vi "Soft_Robot_Model2.vi"() -> ()   [LabVIEW 2015]
uses:
  <vilib>/addons/Control Design/_Model Construction/Model Typedefs.llb/CD State Space Model (MIMO).ctl
  <vilib>/addons/Control Design/_Model Construction/Model Typedefs.llb/CD General Elements.ctl
  <vilib>/Platform/TimedLoop/XDataNode/timing_clust.ctl
  <vilib>/Platform/TimedLoop/XDataNode/nitl_modes.ctl
  <vilib>/Platform/TimedLoop/XDataNode/wakeup.ctl
  <vilib>/addons/Control Design/_Stochastic Systems/Stochastic Systems.llb/Stochastic Systems SubVIs/cd_Stochastic State-Space Model.ctl
  <vilib>/addons/Control Design/_Stochastic Systems/Stochastic Systems.llb/Stochastic Systems SubVIs/cd_Second-Order Statistics Noise Model.ctl
  <vilib>/addons/Control Design/_Model Construction/Model Creation.llb/Model Creation SubVI/cd_Create State Space Model.vi
  <vilib>/Simulation/Estimation/Implementation/NILVSim Discrete Kalman Filter.llb/SIM Disc KF Pred and Corr with Pred Gain with Checking Direct LV.vi
  <vilib>/addons/Control Design/_Implementation/CD State Feedback Controller (Multiple Outputs).vi
  <vilib>/FPGAPlugInAG/myRIO-1900/niLvFpga_Open_myRIO-1900.vi
  <vilib>/rvi/interface/common/dynamic/niFpgaDynamicAddResources.vi
  <vilib>/Utility/error.llb/Error Cluster From Error Code.vi
  <vilib>/rvi/errors/niLvFpgaAdjustHostInterfaceError.vi
  <vilib>/FPGAPlugInAG/Dynamic/niLvFpga_Close_Dynamic.vi
  <vilib>/Simulation/Implementation/XNodeFramework/SimXNode/SimX.xnode
  <vilib>/rvi/interface/nirviOpenFPGA/nirviOpenFPGA.xnode
  FPGA Bitfiles/ACC20115_FPGATarget_CurrentControlle_Dt5vFgOzYtY.lvbitx
  Current Controller.vi
  <vilib>/Platform/TimedLoop/XDataNode/XDataNode.xnode
  <vilib>/rvi/interface/nirviReadWriteControl/nirviReadWriteControl.xnode
  <vilib>/rvi/interface/nirviCloseFPGA/nirviCloseFPGA.xnode
  <vilib>/addons/Control Design/_Model Construction/NI_LinSys_Model Creation.lvlib
  <vilib>/Platform/TimedLoop/XDataNode/XDNodeRunTimeDep.lvlib
  NiFpgaLv.dll
  <vilib>/rvi/interface/Simulation/niFpgaSimulationCallBeginRW.vi
  <vilib>/addons/Control Design/_Implementation/NI_CD_Implementation.lvlib
  <vilib>/addons/Control Design/_Stochastic Systems/NI_CD_Stochastic Systems.lvlib
  <vilib>/addons/Control Design/_Model Construction/NI_LinSys_Model Typedefs.lvlib
panel:
  in  "SP":dbl(slide) scale=0.0..100.0
  in  "Tab Control":enum32{"Outputs", "Inputs"}(tab)
  out "Fusion Data":dbl(graph)
  out "KF Post":dbl[](graph)
  in  "Stop":bool
  out "DAC Inlet Valve 2":i32(graph)
  in  "Current (mA)":i32
  out "Status?":bool
  out "State-Space Model":T1={"properties"={"Model name"="", "Input names"=[], "Output names"=[], "Input Delays"=[], "Output Delays"=[], "Sampling Time"=0.0, "Notes"=""}, "A"=[], "B"=[[3.03e-07], [4.04e-07]], "C"=[], "D"=[], "StateNames"=[], "Transport Delay"=[]} {"Transport Delay" format="%.2f"; "D" format="%#.2g"; "C" format="%#.2g"; "B" format="%#.2g"; "A" format="%#.2g"; "properties"."Sampling Time" format="%#.6p"; "properties"."Output Delays" format="%.4f"; "properties"."Input Delays" format="%.4f"}
  out "KF Gain M(k)":dbl[][](array[numeric])
  in  "A":dbl[][](array[numeric])=[[1.01, -0.1716], [0.001556, 0.9782]] format="%#.5g"
  in  "B":dbl[][](array[numeric]) format="%#.5g"
  in  "C":dbl[][](array[numeric])=[[1.089, -0.03769]] format="%#.5g"
  out "error out":errorcluster
  out "KF Error":errorcluster
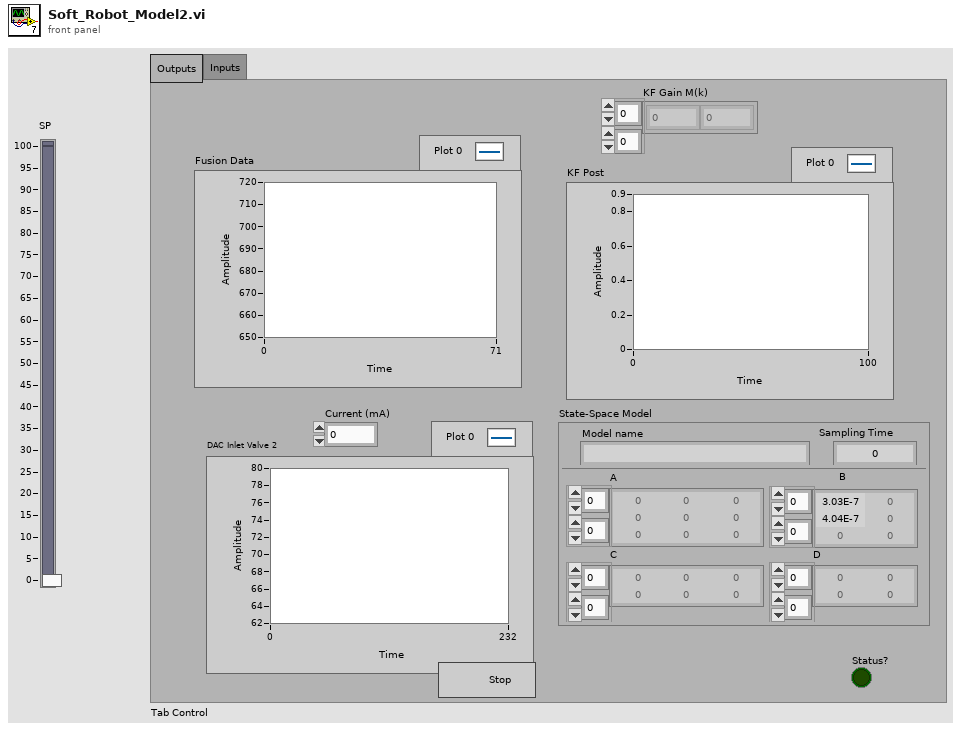
[diagram p1: front panel]
types:
  T1 = typedef "NI_LinSys_Model Typedefs.lvlib/CD State Space Model (MIMO).ctl" = cluster{"properties":T2, "A":dbl[][], "B":dbl[][], "C":dbl[][], "D":dbl[][], "StateNames":string[], "Transport Delay":dbl[][]}
  T2 = typedef "NI_LinSys_Model Typedefs.lvlib/CD General Elements.ctl" = cluster{"Model name":string, "Input names":string[], "Output names":string[], "Input Delays":dbl[], "Output Delays":dbl[], "Sampling Time":dbl, "Notes":string}
  T3 = typedef "NI_CD_Stochastic Systems.lvlib/cd_Second-Order Statistics Noise Model.ctl" = cluster{"Q":dbl[][], "E{w}":dbl[], "E{v}":dbl[], "R":dbl[][], "N":dbl[][]}
  T4 = typedef "NI_CD_Stochastic Systems.lvlib/cd_Stochastic State-Space Model.ctl" = cluster{"Sampling Time (s)":dbl, "G":dbl[][], "B":dbl[][], "A":dbl[][], "C":dbl[][], "D":dbl[][], "H":dbl[][]}
  T5 = typedef "XDNodeRunTimeDep.lvlib/timing_clust.ctl" = cluster{"Expected End [f-1]":u64, "Actual End [f-1]":u64, "Finished Late? [f-1]":bool, "Expected End [i-1]":u64, "Actual End [i-1]":u64, "Finished Late? [i-1]":bool, "Expected Start [i]":u64, "Actual Start [i]":u64, "Expected Start [f]":u64, "Actual Start [f]":u64, "Source Name":string, "Structure Name":string, "Period":i64, "Deadline":i64, "Offset":i64, "Start":i64, "Priority":i32, "Timeout":i32, "Mode":T6, "Wakeup Reason":T7, "Error":errorcluster, "Source Type":string, "Secondary Source Type":string, "Global End Time":u64, "Global Start Time":u64, "Frame Duration":u64, "Iteration Duration":u64, "Assigned CPU":i32, "I/O Scan Engine Mode":u32}
  T6 = typedef "XDNodeRunTimeDep.lvlib/nitl_modes.ctl" = enum32{"No Change", "Process missed periods, maintain original phase", "Discard missed periods, maintain original phase", "Process missed periods, ignore original phase", "Discard missed periods, ignore original phase"}
  T7 = typedef "XDNodeRunTimeDep.lvlib/wakeup.ctl" = enum32{"Normal", "Aborted", "Asynchronous wakeup", "Timing source error", "Timed loop error", "Timeout"}
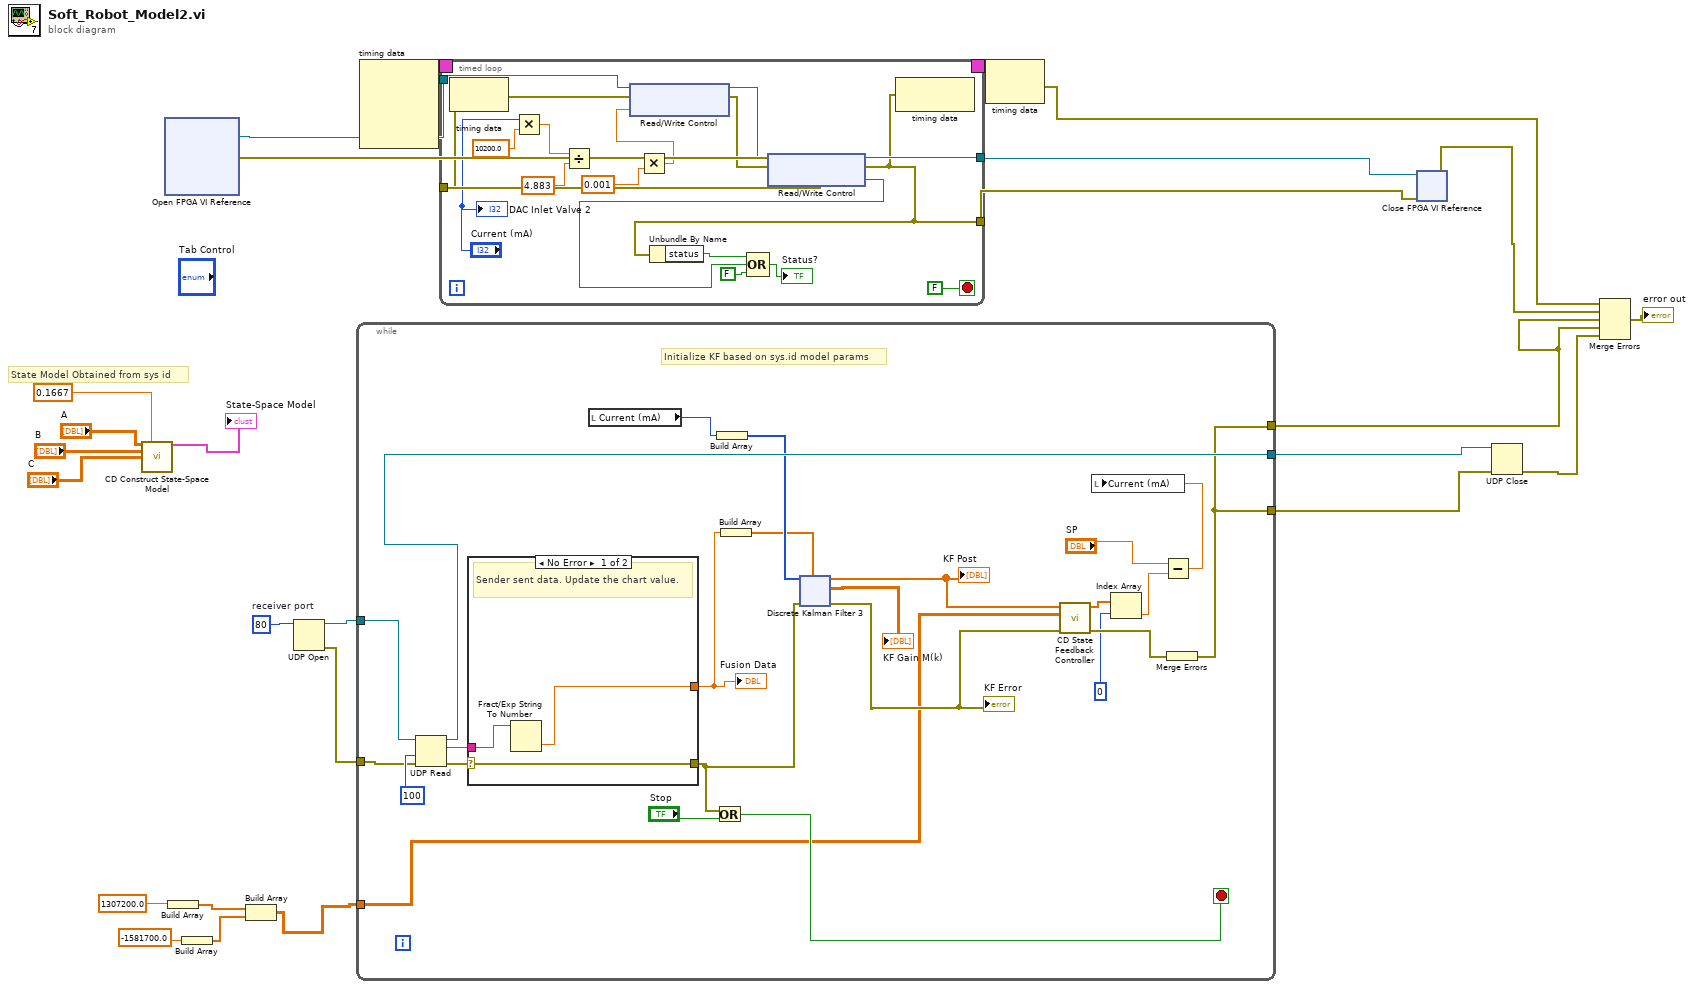
[diagram p0: block diagram]
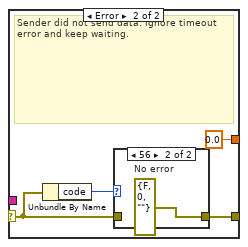
[diagram p2: hidden frame]
diagram:
  w25 = u16 80  # receiver port
  # "State Model Obtained from sys id"
  n1 = call-poly <vilib>:"CD Construct State-Space Model.vi"("A"="A", "Sampling Time (s)"=0.1667, "B"="B", "C"="C") -> ("State-Space Model"=→"State-Space Model":T1)  [unwired: 10 in, 1 out]
  n2 = xnode "Open FPGA VI Reference"() -> ("FPGA VI Reference Out"=w20:refnum<k20>, "error out"=w19:errorcluster)  [unwired: 2 in]
  n3 = Build Array(1307200.0 ("element")) -> (w4:dbl[])
  n4 = Build Array(-1581700.0 ("element")) -> (w3:dbl[])
  n5 = Build Array(w4, w3) -> (w2:dbl[][])
  n6 = UDP Open(11:w25) -> (port=w24:refnum<k16>, 0:w23:errorcluster)  [unwired: 4 in, 1 out]
  n7 = while {
    tunnel: [w33] -> w1
    tunnel: w24 -> [w45]
    tunnel: w23 -> [w44]
    tunnel: [w42] -> w22
    tunnel: [w33] -> w16
    tunnel: w2 -> [w32]
    stop <- w43 stop-if-true
    # "Initialize KF based on sys.id model params"
    n8 = UDP Read(connection ID=w45, timeout ms (25000)=100, 8:w44) -> (data out=w47:string, error out=w46:errorcluster, 3:w42:refnum<k16>)  [unwired: 3 out]
    n9 = case shown="No Error" w46 {
      selector: w46 -> [w52 w56]
      tunnel: w47 -> [w53 _]
      tunnel: [w52 w55] -> w27
      tunnel: [w51 0.0] -> w37
      frame No Error {
        # "Sender sent data. Update the chart value."
        n10 = Fract/Exp String To Number(string=w53) -> (number=w51:dbl)  [unwired: 3 in, 1 out]
      }
      frame Error {
        # "Sender did not send data. Ignore timeout error and keep waiting."
        n11 = Unbundle By Name(w56) -> ("code"=w57:i32)
        n12 = case shown="56" w57 {
          tunnel: w56 -> [w58 _]
          tunnel: [w58 w59] -> w55
          frame Default {
          }
          frame 56 {
            w59 = errorcluster {"status"=FALSE, "code"=0, "source"=""}  # No error
          }
        }
      }
    }
    "Fusion Data" <- w37
    n13 = local read "Current (mA)"() -> (w50:i32)
    n14 = Or(x=w27, y="Stop") -> (x .or. y?=w43:bool)
    n15 = Build Array ("Build Array 5")(w50) -> (w38:i32[])
    n16 = Build Array ("Build Array 6")(w37) -> (w36:dbl[])
    n17 = xnode ("Discrete Kalman Filter 3")("input u(k)"=w38, "Output y(k)"=w36, "error in (no error)"=w27) -> ("Corrected State Estimate xhat(k|k)"=w28:dbl[], "Kalman Filter Gain M(k)"=→"KF Gain M(k)":dbl[][], "error out"=w39:errorcluster)  [unwired: 5 out]
    "KF Post" <- w28
    "KF Error" <- w39
    n18 = call-poly <vilib>:"CD State Feedback Controller.vi"("error in (no error)"=w39, "Controller Gain"=w32, "States"=w28) -> ("error out"=w40:errorcluster, "Controller Action"=w35:dbl[])  [unwired: 7 in]
    n19 = Index Array(array=w35, index=0) -> (element=w31:dbl)
    n20 = Subtract(x="SP", y=w31) -> (x-y=w30:dbl)
    n21 = local write "Current (mA)"(w30) -> ()
    n22 = Merge Errors(w40) -> (w33:errorcluster)
  }
  n23 = node-c288() -> (w18:T5)  [unwired: 4 in]
  n24 = timed-loop {
    tunnel: w20 -> [w92]
    tunnel: w19 -> [w77]
    tunnel: [w76] -> w10
    tunnel: [w85] -> w26
    timing: w18 -> [_]
    timing-out: [_] -> w17
    stop <- FALSE stop-if-true
    n25 = node-c288() -> ()  [unwired: 1 in, 1 out]
    n26 = Multiply(x="Current (mA)", y=10200.0) -> (x*y=w80:dbl)
    n27 = Divide(x=w80, y=4.883) -> (x/y=w83:dbl)
    n28 = Multiply(x=w83, y=0.001) -> (x*y=w79:dbl)
    n29 = xnode "Read/Write Control"("FPGA VI Reference In"=w92, "error in"=w77, "DAC Inlet Valve"=w79) -> ("FPGA VI Reference Out"=w91:refnum<k20>, "error out"=w90:errorcluster)
    n30 = xnode "Read/Write Control"("FPGA VI Reference In"=w91, "error in"=w90) -> ("FPGA VI Reference Out"=w85:refnum<k20>, "error out"=w76:errorcluster, "Inlet Overflow?"=w86:bool)
    n31 = Unbundle By Name(w76) -> ("status"=w88:bool)
    n32 = Compound Arithmetic op=OR(w88, w86, FALSE ("value")) -> (→"Status?":bool)
    n33 = node-c288(w76) -> ()  [unwired: 1 out]
    "DAC Inlet Valve 2" <- "Current (mA)"
  }
  n34 = node-c288(w17) -> (w7:errorcluster)
  n35 = xnode "Close FPGA VI Reference"("FPGA VI Reference In"=w26, "error in"=w10) -> ("error out"=w8:errorcluster)
  n36 = UDP Close(connection ID=w22, 8:w16) -> (error out=w9:errorcluster)  [unwired: 1 out]
  n37 = Merge Errors(w7, w8, w1, w1, w9) -> (→"error out":errorcluster)
